vi "MAUI.GetPrivateEvents.vi"(8 "error in (no error)":errorcluster, 11 "MAUI":refnum<class "MAUI.lvclass">) -> (0 "error out":errorcluster, 2 "Private Events":T1, 3 "MAUI out":refnum<class "MAUI.lvclass">)   [LabVIEW 2019, in "MAUI.lvclass"]
doc: "---------------------------------------------------------------\nJKI State Machine Objects™\nhttp://jki.net/state-machine-objects/\nCopyright (C) 2005-2015, JKI <info@jki.net>\nALL RIGHTS RESERVEDJKI State Machine Objects (SMO) 1.0.0.4\nJKI - JKI\nCopyright (c) 2015, JKI"
uses:
  MAUI.lvclass
  Typedefs/PrivateEvents--Cluster.ctl
  Typedefs/PanelData.ctl
  Typedefs/PrivateEvents--MAUI.SetEmbedded.ctl
  Typedefs/PrivateEvents--MAUI.GetEmbedded.ctl
  Typedefs/PrivateEvents--MAUI.SetPanelData.ctl
  Typedefs/PrivateEvents--MAUI.GetPanelData.ctl
  Typedefs/PrivateEvents--MAUI.UpdatePanel.ctl
  <userlib>/LevyLab/Embedded UI/Embedded UI/Embedded UI.lvclass
  Typedefs/PrivateEvents--MAUI.OpenSubpanel.ctl
  Typedefs/PrivateEvents--MAUI.GetDefaultSubpanel.ctl
  Typedefs/DefaultSubpanel.ctl
  Typedefs/PrivateEvents--MAUI.SetDefaultSubpanel.ctl
panel:
  # "For instructions on how to use the JKI State Machine Objects, examples and video tutorials, visit:\nhttp://jki.net/state-machine-objects/\n\nJKI State Machine Objects™\nhttp://jki.net/state-machine-objects/\nCopyright (C) 2005-2015, JKI <info@jki.net>\nALL RIGHTS RESERVED"
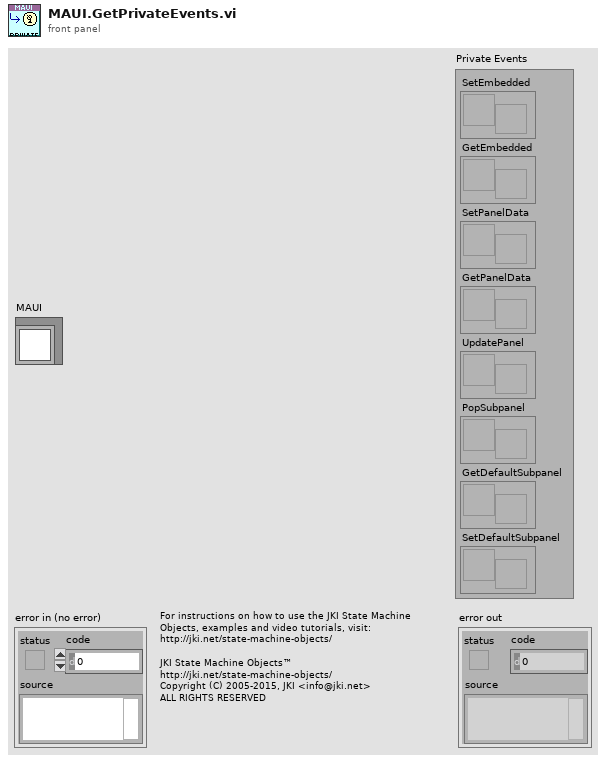
[diagram p1: front panel]
types:
  T1 = typedef "MAUI.lvclass/PrivateEvents--Cluster.ctl" = cluster{"SetEmbedded":refnum<user-event>, "GetEmbedded":refnum<user-event>, "SetPanelData":refnum<user-event>, "GetPanelData":refnum<user-event>, "UpdatePanel":refnum<user-event>, "PopSubpanel":refnum<user-event>, "GetDefaultSubpanel":refnum<user-event>, "SetDefaultSubpanel":refnum<user-event>}
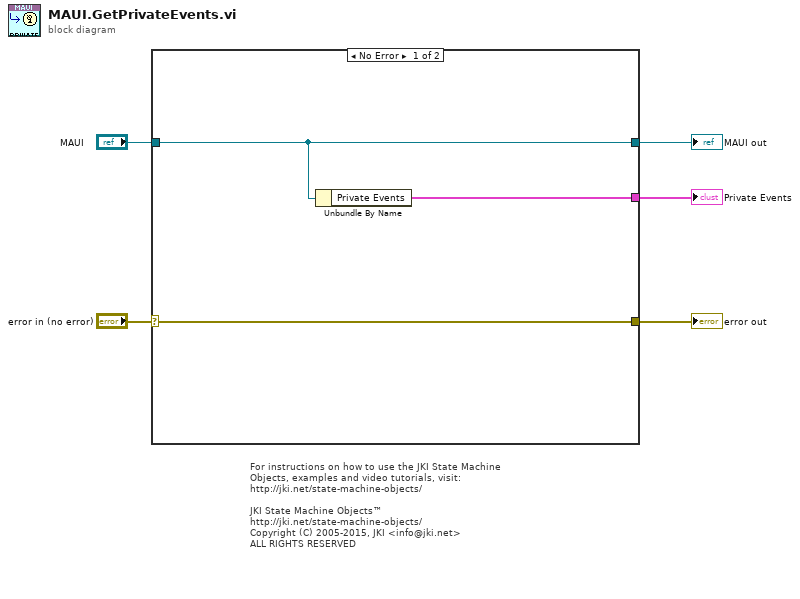
[diagram p0: block diagram]
diagram:
  # "For instructions on how to use the JKI State Machine Objects, examples and video tutorials, visit:\nhttp://jki.net/state-machine-objects/\n\nJKI State Machine Objects™\nhttp://jki.net/state-machine-objects/\nCopyright (C) 2005-2015, JKI <info@jki.net>\nALL RIGHTS RESERVED"
  n1 = case shown="No Error" "error in (no error)" {
    selector: "error in (no error)" -> [w8 w9]
    tunnel: "MAUI" -> [w7 w10]
    tunnel: [w8 w9] -> w4
    tunnel: [w7 w10] -> w3
    tunnel: [w6 _] -> w1
    frame No Error {
      n2 = Unbundle By Name(w7) -> ("Private Events"=w6:T1)
    }
    frame Error {
    }
  }
  "error out" <- w4
  "MAUI out" <- w3
  "Private Events" <- w1
